vi "Page Help.vi"() -> ()   [LabVIEW 2018, in "Main.lvlib"]
uses:
  Main.lvlib
  Exit/Exit.lvlib
  Help/Help.lvlib
  Help/Action.ctl
panel:
  in  "Search":string caption="Help"
  in  "Help Lbx":i32(listbox)=-1
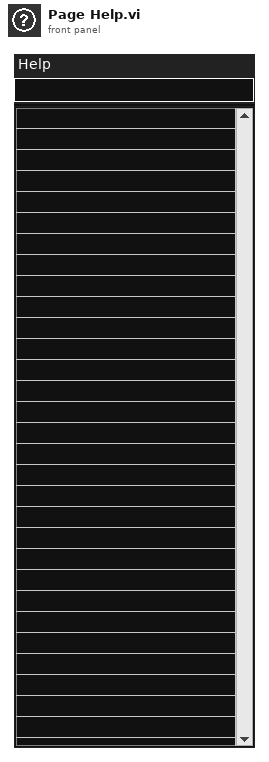
[diagram p1: front panel]
types:
  T1 = typedef "Help.lvlib/Action.ctl" = enum8{"noop", "new", "init", "close", "load", "render", "filter", "topic"}
  T2 = cluster{"Search":refnum<vi>, "Tree":refnum<vi>, "Picture":refnum<vi>}
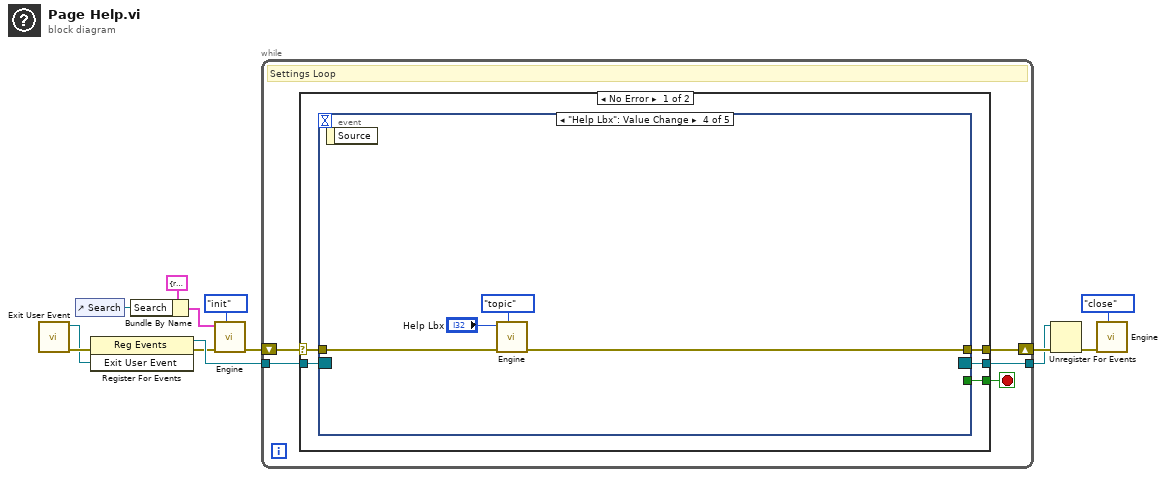
[diagram p0: block diagram]
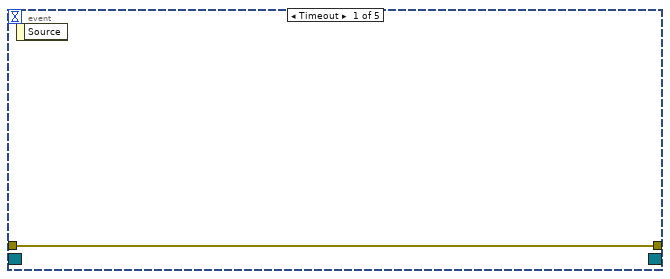
[diagram p2: hidden frame]
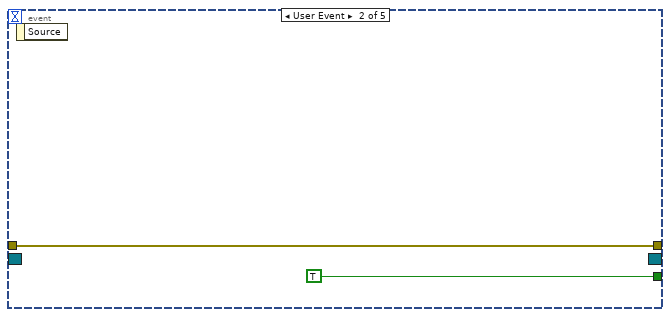
[diagram p3: hidden frame]
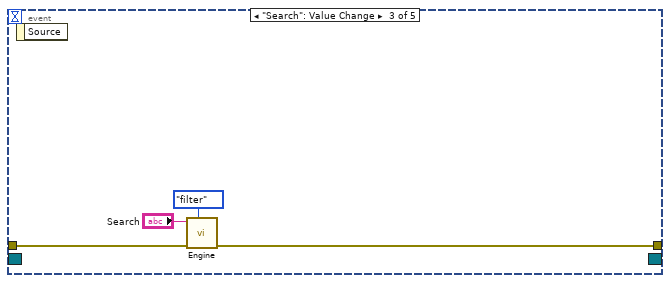
[diagram p4: hidden frame]
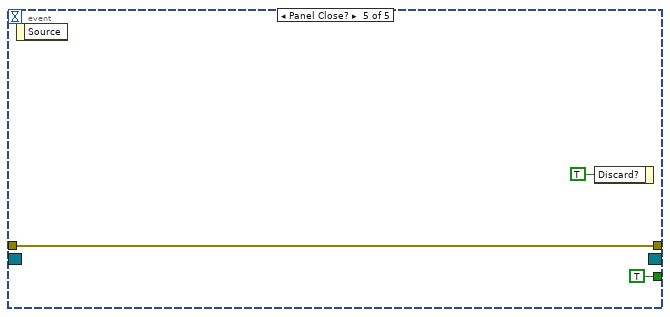
[diagram p5: hidden frame]
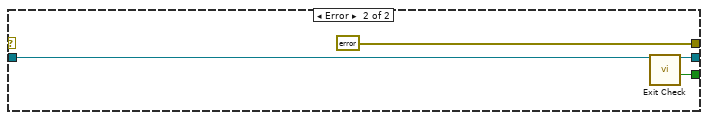
[diagram p6: hidden frame]
diagram:
  n1 = call "Exit User Event.vi"() -> ("error out"=w13:errorcluster, "Exit User Event"=w12:refnum<user-event>)  [unwired: 10 in]
  n2 = control-ref of="Search"() -> (w6:refnum<vi>)
  n3 = register-events(error in=w13, w12) -> (reference out=w11:refnum<event-registration>, error out=w2:errorcluster)  [unwired: 1 in]
  n4 = Bundle By Name(cluster=T2 {"Search"=refnum, "Tree"=refnum, "Picture"=refnum} ("Init"), "Search"=w6) -> (w5:T2)
  n5 = call "Engine.vi"("Action"=Action."init", "error in (no error)"=w2, "Variant in"=w5) -> ("error out"=w1:errorcluster)  [unwired: 7 in, 1 out]
  n6 = while {
    tunnel: w11 -> [w17]
    shift-right: [w16] -> w10
    shift-left: w1 -> [w18]
    tunnel: [w14] -> w9
    stop <- w15 stop-if-true
    # "Settings Loop"
    n7 = case shown="No Error" w18 {
      selector: w18 -> [w23 _]
      tunnel: w17 -> [w22 w38]
      tunnel: [w21 errorcluster {"status"=FALSE, "code"=0, "source"=""} ("error IO")] -> w16
      tunnel: [w19 w39] -> w15
      tunnel: [w20 w38] -> w14
      frame No Error {
        n8 = event shown="[3] \"Help Lbx\": Value Change" {
          selector: w22 -> [_ _ _ _ _]
          dyn-events: [_ _ _ _ _] -> w20
          timeout: _ -> [_ _ _ _ _]
          tunnel: w23 -> [w24 w26 w29 w33 w37]
          tunnel: [w24 w26 w28 w32 w37] -> w21
          tunnel: [_ TRUE _ _ TRUE] -> w19
          event Timeout {
            n9 = event-data() -> ()  [unwired: 1 in, 1 out]
          }
          event User Event {
            n10 = event-data() -> ()  [unwired: 1 in, 1 out]
          }
          event "Search": Value Change {
            n11 = event-data() -> ()  [unwired: 1 in, 1 out]
            n12 = call "Engine.vi"("Action"=Action."filter", "error in (no error)"=w29, "Variant in"="Search") -> ("error out"=w28:errorcluster)  [unwired: 7 in, 1 out]
          }
          event "Help Lbx": Value Change {
            n13 = event-data() -> ()  [unwired: 1 in, 1 out]
            n14 = call "Engine.vi"("Action"=Action."topic", "error in (no error)"=w33, "Variant in"="Help Lbx") -> ("error out"=w32:errorcluster)  [unwired: 7 in, 1 out]
          }
          event Panel Close? {
            n15 = event-data() -> ()  [unwired: 1 in, 1 out]
            n16 = event-data("Discard?"=TRUE) -> ()  [unwired: 1 in, 1 out]
          }
        }
      }
      frame Error {
        n17 = call "Exit Check.vi"() -> ("Exit?"=w39:bool)  [unwired: 10 in, 1 out]
      }
    }
  }
  n18 = Unregister For Events(event registration refnum=w9, error in=w10) -> (error out=w3:errorcluster)
  n19 = call "Engine.vi"("Action"=Action."close", "error in (no error)"=w3) -> ()  [unwired: 8 in, 2 out]
